vi "InitMH_UIThread.vi"(8 "error in (no error)":errorcluster, 9 "Mode":T2 items=["HIST"=0, "T2"=2, "T3"=3], 10 "refsource":T1, 11 "Library Version":string="1.0") -> (0 "error out":errorcluster, 2 "Init Info":T3, 3 "DevIdx":i32)   [LabVIEW 2010]
uses:
  MH_InitInfo.ctl
  MH_MeasMode.ctl
  MH_RefSource.ctl
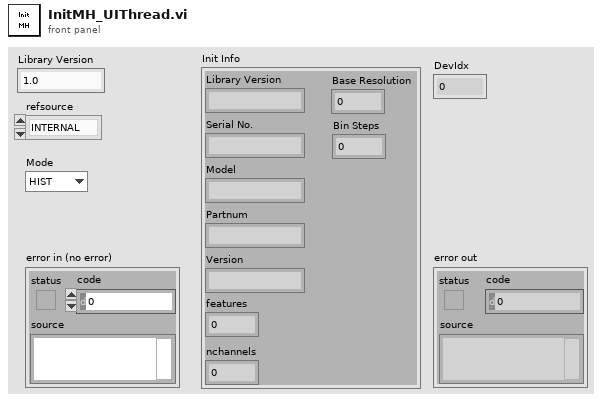
[diagram p1: front panel]
types:
  T1 = typedef "MH_RefSource.ctl" = enum16{"INTERNAL", "EXTERNAL_10MHZ", "WR_MASTER_GENERIC", "WR_SLAVE_GENERIC", "WR_GRANDM_GENERIC", "EXTN_GPS_PPS", "EXTN_GPS_PPS_UART", "WR_MASTER_MHARP", "WR_SLAVE_MHARP", "WR_GRANDM_MHARP"}
  T2 = typedef "MH_MeasMode.ctl" = i32
  T3 = typedef "MH_InitInfo.ctl" = cluster{"Library Version":string, "Serial No.":string, "Model":string, "Partnum":string, "Version":string, "features":i32, "nchannels":i32, "Base Resolution":dbl, "Bin Steps":i32}
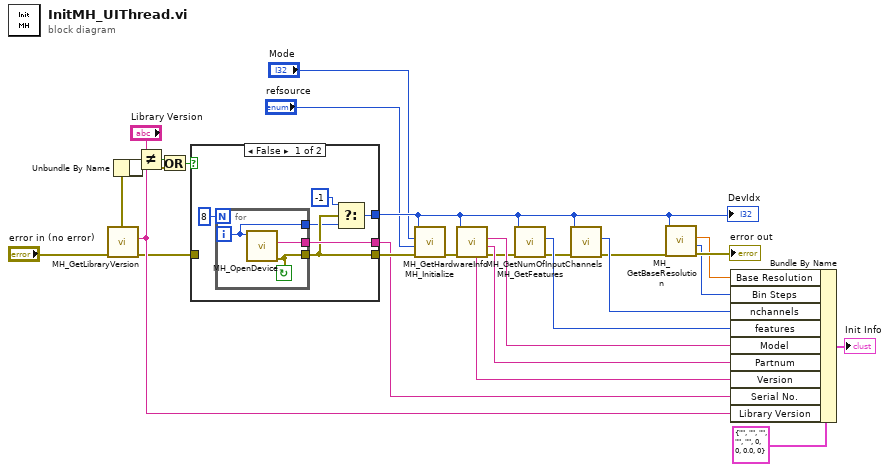
[diagram p0: block diagram]
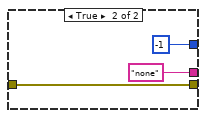
[diagram p2: hidden frame]
diagram:
  n1 = call "MH_GetLibraryVersion.vi"("error in (no error)"="error in (no error)") -> ("error out"=w7:errorcluster, "Version"=w15:string)  [unwired: 8 in, 1 out]
  n2 = Not Equal?(x="Library Version", y=w15) -> (x != y?=w25:bool)
  n3 = Or(x=w25) -> (y=w1:errorcluster, x .or. y?=w24:bool)
  n4 = Unbundle By Name(w7, w1) -> ()
  n5 = case shown="False" w24 {
    tunnel: [w28 -1 ("return type")] -> w6
    tunnel: [w31 "none" ("serial")] -> w17
    tunnel: [w30 w36] -> w23
    tunnel: w7 -> [_ w36]
    frame False {
      n6 = for {
        N: 8 -> [_]
        tunnel: [w34] -> w30
        tunnel: [w33] -> w31
        tunnel: [w35] -> w29
        i -> [w35]
        stop <- w34 continue-if-true
        n7 = call "MH_OpenDevice.vi"("devidx"=w35) -> ("error out"=w34:errorcluster, "serial"=w33:string)  [unwired: 8 in, 1 out]
      }
      n8 = Select(t=-1, s=w30, f=w29) -> (s? t:f=w28:i32)
    }
    frame True {
    }
  }
  "DevIdx" <- w6
  n9 = call "MH_Initialize.vi"("error in (no error)"=w23, "refsource"="refsource", "mode"="Mode", "devidx"=w6) -> ("error out"=w22:errorcluster)  [unwired: 6 in, 1 out]
  n10 = call "MH_GetHardwareInfo.vi"("error in (no error)"=w22, "devidx"=w6) -> ("error out"=w13:errorcluster, "Partnum"=w20:string, "Model"=w21:string, "Version"=w19:string)  [unwired: 5 in, 1 out]
  n11 = call "MH_GetFeatures.vi"("error in (no error)"=w13, "devidx"=w6) -> ("error out"=w5:errorcluster, "features"=w18:i32)  [unwired: 7 in, 1 out]
  n12 = call "MH_GetNumOfInputChannels.vi"("error in (no error)"=w5, "devidx"=w6) -> ("error out"=w2:errorcluster, "nchannels"=w12:i32)  [unwired: 7 in, 1 out]
  n13 = call "MH_GetBaseResolution.vi"("error in (no error)"=w2, "devidx"=w6) -> ("error out"=→"error out":errorcluster, "binsteps"=w10:i32, "resolution"=w9:dbl)  [unwired: 6 in, 1 out]
  n14 = Bundle By Name(cluster=T3 {"Library Version"="", "Serial No."="", "Model"="", "Partnum"="", "Version"="", "features"=0, "nchannels"=0, "Base Resolution"=0.0, "Bin Steps"=0} ("Init"), "Base Resolution"=w9, "Bin Steps"=w10, "nchannels"=w12, "features"=w18, "Model"=w21, "Partnum"=w20, "Version"=w19, "Serial No."=w17, "Library Version"=w15) -> (→"Init Info":T3)
